vi "Nearly Equal.vi"(8 "tolerance":dbl=0.1, 10 "y":dbl, 11 "x":dbl) -> (3 "nearly equal":bool)   [LabVIEW 2011]
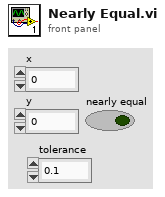
[diagram p1: front panel]
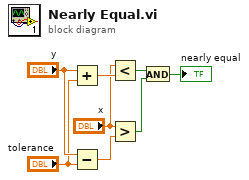
[diagram p0: block diagram]
diagram:
  n1 = Add(x="y", y="tolerance") -> (x+y=w5:dbl)
  n2 = Subtract(x="y", y="tolerance") -> (x-y=w4:dbl)
  n3 = Less?(x="x", y=w5) -> (x < y?=w8:bool)
  n4 = Greater?(x="x", y=w4) -> (0:w7:bool)
  n5 = And(x=w8, y=w7) -> (x .and. y?=→"nearly equal":bool)
